vi "Add State String to Row Index Mapping.vi"(8 "error in (no error)":errorcluster, 9 "Row Index":i32, 10 "State String":string, 11 "StateMachine in":refnum<class "StateMachine.lvclass">) -> (0 "error out":errorcluster, 2 "replaced?":bool, 3 "StateMachine out":refnum<class "StateMachine.lvclass">)   [LabVIEW 2019, in "State Machine.lvlib" / "StateMachine.lvclass"]
doc: "This VI translates a string into a row index in the state machine table."
uses:
  StateMachine.lvclass
  StateMachine.lvclass/StateMachine.ctl
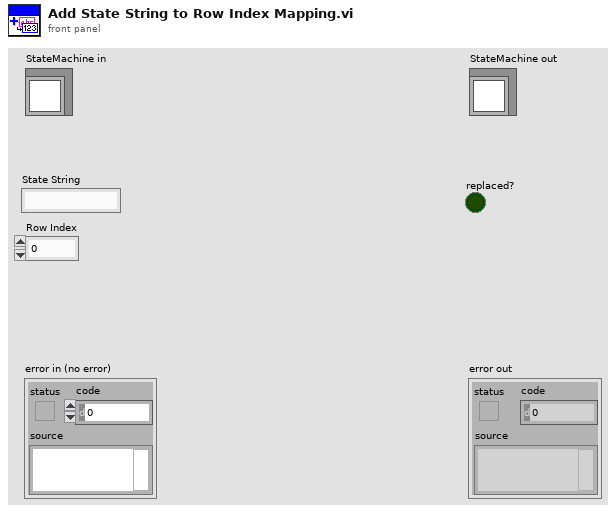
[diagram p1: front panel]
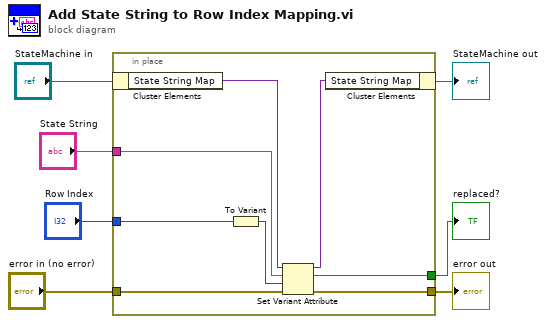
[diagram p0: block diagram]
diagram:
  n1 = in-place {
    in-place-border: "State String" -> [w14]
    in-place-border: "Row Index" -> [w13]
    in-place-border: "error in (no error)" -> [w11]
    in-place-border: [w10] -> w1
    in-place-border: [w8] -> w6
    n2 = in-place-cluster #1("StateMachine in") -> ("State String Map"=w15:variant)
    n3 = To Variant(anything=w13) -> (Variant=w12:variant)
    n4 = Set Variant Attribute(Variant=w15, name=w14, value=w12, error in=w11) -> (Variant out=w9:variant, replaced=w10:bool, error out=w8:errorcluster)
    n5 = in-place-cluster #1("State String Map"=w9) -> (→"StateMachine out":refnum<class "StateMachine.lvclass">)
  }
  "error out" <- w6
  "replaced?" <- w1
